vi "HXG2boolselcFGV.vi"(7 "BoolselecFGV":T2, 8 "error in (no error)":errorcluster, 11 "Boolean Selections":T1) -> (0 "error out":errorcluster, 3 "BoolSelecOut":T1)   [LabVIEW 2012]
uses:
  HXG2boolselec.ctl
  Controls/HXG2_BooleanSelections.ctl
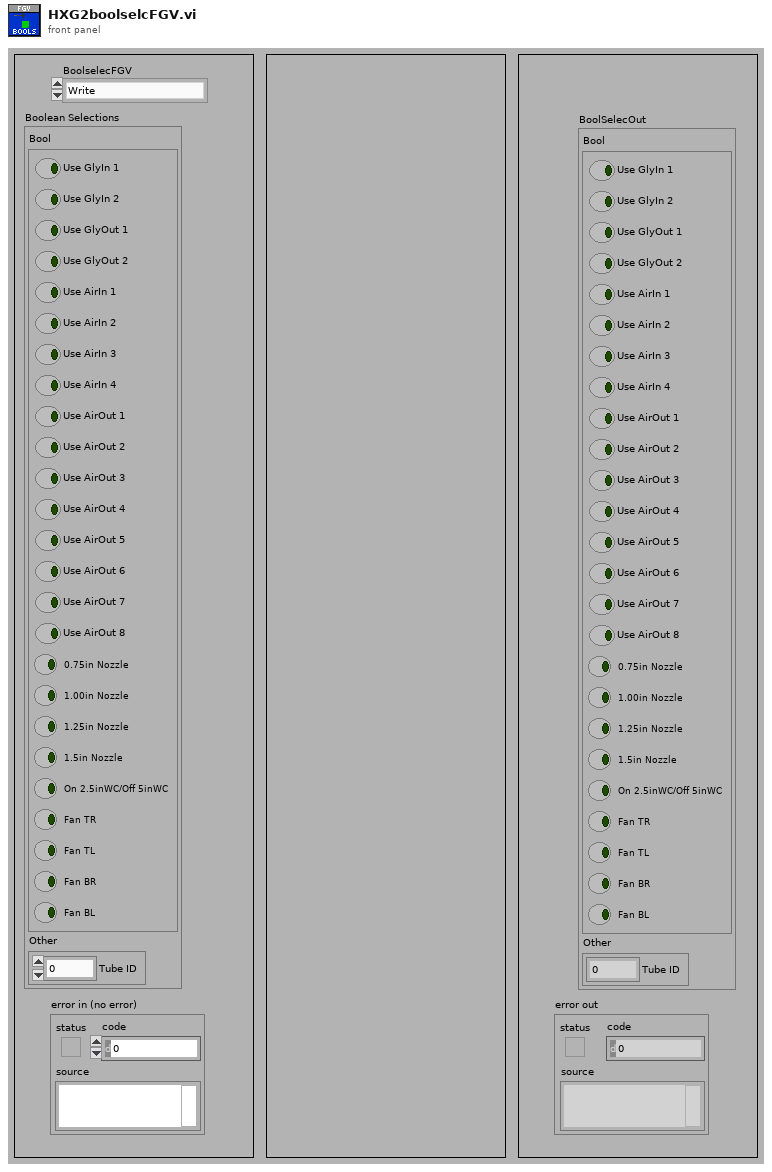
[diagram p1: front panel]
types:
  T1 = typedef "HXG2_BooleanSelections.ctl" = cluster{"Bool":cluster{"Use GlyIn 1":bool, "Use GlyIn 2":bool, "Use GlyOut 1":bool, "Use GlyOut 2":bool, "Use AirIn 1":bool, "Use AirIn 2":bool, "Use AirIn 3":bool, "Use AirIn 4":bool, "Use AirOut 1":bool, "Use AirOut 2":bool, "Use AirOut 3":bool, "Use AirOut 4":bool, "Use AirOut 5":bool, "Use AirOut 6":bool, "Use AirOut 7":bool, "Use AirOut 8":bool, "0.75in Nozzle":bool, "1.00in Nozzle":bool, "1.25in Nozzle":bool, "1.5in Nozzle":bool, "On 2.5inWC/Off 5inWC":bool, "Fan TR":bool, "Fan TL":bool, "Fan BR":bool, "Fan BL":bool}, "Other":cluster{"Tube ID":dbl}}
  T2 = typedef "HXG2boolselec.ctl" = enum16{"Write", "Pass"}
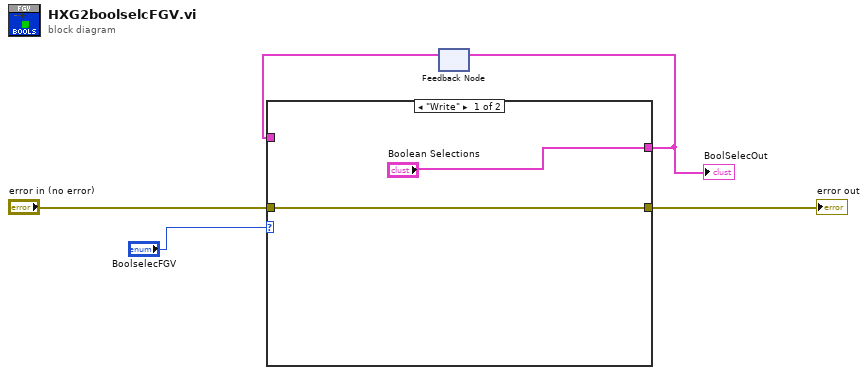
[diagram p0: block diagram]
diagram:
  n1 = feedback #1() -> (w2:T1)  [unwired: 1 in]
  n2 = case shown="\"Write\"" "BoolselecFGV" {
    tunnel: "error in (no error)" -> [w7 w8]
    tunnel: [w7 w8] -> w4
    tunnel: ["Boolean Selections" w9] -> w3
    tunnel: w2 -> [_ w9]
    frame "Write" {
    }
    frame "Pass" {
    }
  }
  "error out" <- w4
  "BoolSelecOut" <- w3
  n3 = feedback-in #1(w3) -> ()
